vi "Get Package Paths.vi"(5 "ms timeout (-1)":i32=-1, 8 "GLue in":refnum<class "class.GLue.lvclass">, 11 "error in":errorcluster) -> (0 "GLue out":refnum<class "class.GLue.lvclass">, 1 "Lpaths":string[](array[string]), 2 "Cpaths":string[](array[string]), 3 "error out":errorcluster)   [LabVIEW 2014, in "GLue.lvlib"]
doc: "Get the paths that are currently being used to search for Lua and C modules, see http://www.lua.org/manual/5.2/manual.html#pdf-package.searchpath for further details.\n\n<B>Parameter(s) </B>\n-----------------\n\n- <B>GLue in:</B> Reference to the GLue instance.\n\n- <B>ms timeout (-1):</B> The time to wait for the GLue reference to become available. A value of '-1' specifies an infinite timeout.\n\n- <B>error in:</B> Describes error conditions that occur before this VI runs. This input provides standard error in functionality. \n\n- <B>GLue out:</B> Reference to the GLue instance.\n\n- <B>Lpaths:</B> An array of possible paths to Lua script modules.\n\n- <B>Cpaths:</B> An array of possible paths to compiled C modules.\n\n- <B>error out:</B> Contains error information. This output provides standard error out functionality."
uses:
  GLue.lvlib
  Private/Class/class.GLue.lvclass
panel:
  # "Input"
  # "Output"
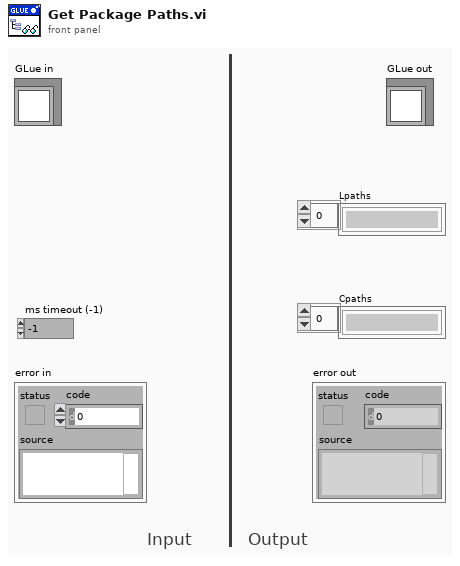
[diagram p1: front panel]
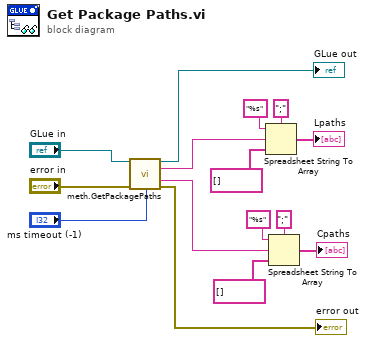
[diagram p0: block diagram]
diagram:
  n1 = call "meth.GetPackagePaths.vi"("class.GLue in"="GLue in", "error in"="error in", "ms timeout (-1)"="ms timeout (-1)") -> ("class.GLue out"=→"GLue out":refnum<class "class.GLue.lvclass">, "Lpaths"=w1:string, "Cpaths"=w7:string, "error out"=→"error out":errorcluster)  [unwired: 9 in]
  n2 = Spreadsheet String To Array(delimiter (Tab)=";", format string="%s", spreadsheet string=w1, array type (2D Dbl)=string[] []) -> (array=→"Lpaths":string[])
  n3 = Spreadsheet String To Array(delimiter (Tab)=";", format string="%s", spreadsheet string=w7, array type (2D Dbl)=string[] []) -> (array=→"Cpaths":string[])
